vi "Grab Image from Android.vi"(8 "error in (no error)":errorcluster, 10 "url":string="192.168.0.12:8080/shot.jpg", 11 "client handle":T1) -> (0 "error out":errorcluster, 2 "data out":string, 3 "client handle out":T1)   [LabVIEW 2012]
uses:
  <vilib>/httpClient/ClientHandle.ctl
  <vilib>/httpClient/LabVIEWHTTPClient.lvlib
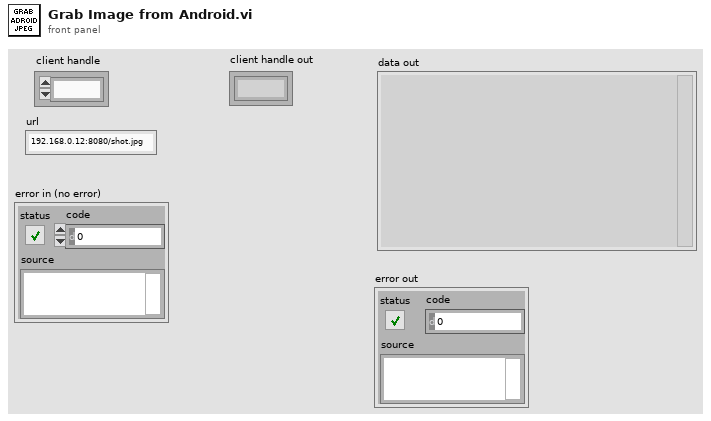
[diagram p1: front panel]
types:
  T1 = typedef "LabVIEWHTTPClient.lvlib/ClientHandle.ctl" = refnum<k1>
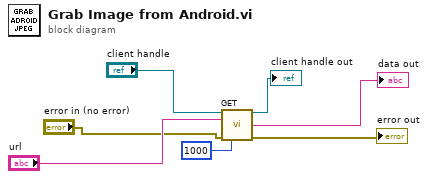
[diagram p0: block diagram]
diagram:
  n1 = call <vilib>:"GET.vi"("client handle"="client handle", "url"="url", "error in (no error)"="error in (no error)", "timeout (10000)"=1000) -> ("client handle out"=→"client handle out":T1, "body"=→"data out":string, "error out"=→"error out":errorcluster)  [unwired: 8 in, 1 out]
